vi "Set_Emission.vi"(8 "error in (no error)":errorcluster, 10 "Emission status":bool, 11 "NKT in":refnum<class "NKT_Extreme.lvclass">) -> (0 "error out":errorcluster, 3 "NKT out":refnum<class "NKT_Extreme.lvclass">)   [LabVIEW 2020, in "NKT_Extreme.lvclass"]
uses:
  <instrlib>/Classes/Laser/NKT/NKT_Extreme.lvclass
  <instrlib>/NKTP_API/NKTP_API.lvlib
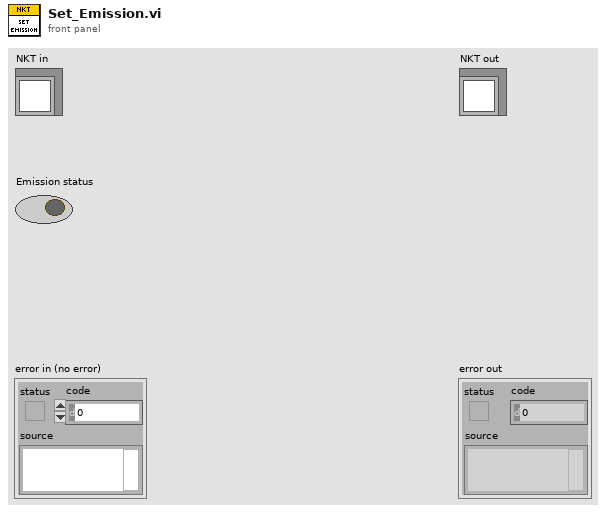
[diagram p1: front panel]
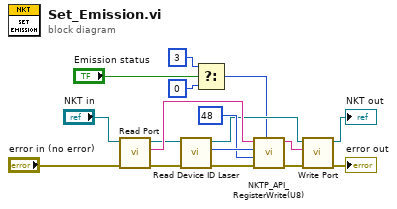
[diagram p0: block diagram]
diagram:
  n1 = call-dynamic "Read Port.vi"("error in (no error)"="error in (no error)", "NKT in"="NKT in") -> ("error out"=w14:errorcluster, "Port"=w17:string, "NKT out"=w15:refnum<class "NKT_Extreme.lvclass">)  [unwired: 7 in]
  n2 = call-dynamic "Read Device ID Laser.vi"("error in (no error)"=w14, "NKT in"=w15) -> ("error out"=w10:errorcluster, "Device ID Laser"=w12:u8, "NKT out"=w9:refnum<class "NKT_Extreme.lvclass">)  [unwired: 7 in]
  n3 = Select(t=u8 3 ("value"), s="Emission status", f=u8 0) -> (s? t:f=w1:u8)
  n4 = call <instrlib>:"NKTP_API_RegisterWrite(U8).vi"("value"=w1, "error in"=w10, "regId"=u8 48, "devId"=w12, "portname"=w17) -> ("error out"=w8:errorcluster, "portname out"=w7:string)  [unwired: 5 in]
  n5 = call-dynamic "Write Port.vi"("error in (no error)"=w8, "Port"=w7, "NKT in"=w9) -> ("error out"=→"error out":errorcluster, "NKT out"=→"NKT out":refnum<class "NKT_Extreme.lvclass">)  [unwired: 7 in]
